vi "Set 1D Array Double Complex.vi"(5 "use temporary file? (F)":bool, 7 "column vector?":bool, 8 "error in":errorcluster, 9 "value":cdb[](array[numeric]), 10 "variable name":string, 11 "GOLPI ref. in":T1={"pipe handle"={"lv_proc.dll file path"=path "", "process instance handle"=[], "debug mode"=FALSE, "debug data"=[]}, "fast read timeout [ms]"=500, "fast read settle time [ms]"=10, "fast read to multiple [ms]"=1, "max elements per input line"=100, "slow read timeout [ms]"=5000, "stdin double format specifier"="%_16e", "max elements per stdout output column"=100, "console mode bitstream"=FALSE, "bitstream first read timeout [ms]"=1000, "bitstream read timeout [ms]"=50, "struct transfer possible"=FALSE, "matlab mode"=FALSE, "var pipe write timeout [ms]"=5000, "variable pipe mode"=FALSE, "variable pipe buffer size [Bytes]"=10000000, "variable pipe block size [Bytes]"=1000000} {"variable pipe block size [Bytes]" format="%.0p"; "variable pipe buffer size [Bytes]" format="%.0p"}) -> (0 "error out":errorcluster, 3 "GOLPI ref. out":T1={"pipe handle"={"lv_proc.dll file path"=path "", "process instance handle"=[], "debug mode"=FALSE, "debug data"=[]}, "fast read timeout [ms]"=500, "fast read settle time [ms]"=10, "fast read to multiple [ms]"=1, "max elements per input line"=100, "slow read timeout [ms]"=5000, "stdin double format specifier"="%_16e", "max elements per stdout output column"=100, "console mode bitstream"=FALSE, "bitstream first read timeout [ms]"=1000, "bitstream read timeout [ms]"=50, "struct transfer possible"=FALSE, "matlab mode"=FALSE, "var pipe write timeout [ms]"=5000, "variable pipe mode"=FALSE, "variable pipe buffer size [Bytes]"=10000000, "variable pipe block size [Bytes]"=1000000} {"variable pipe block size [Bytes]" format="%.0p"; "variable pipe buffer size [Bytes]" format="%.0p"})   [LabVIEW 2020, in "GOLPI library.lvlib"]
doc: "Part of polymorph Set Variable.vi"
uses:
  GOLPI library.lvlib
  Public/GOLPI reference Type Def.ctl
  LV Process source distribution/Pipe Handle.ctl
  LV Process source distribution/LV Process library.lvlib
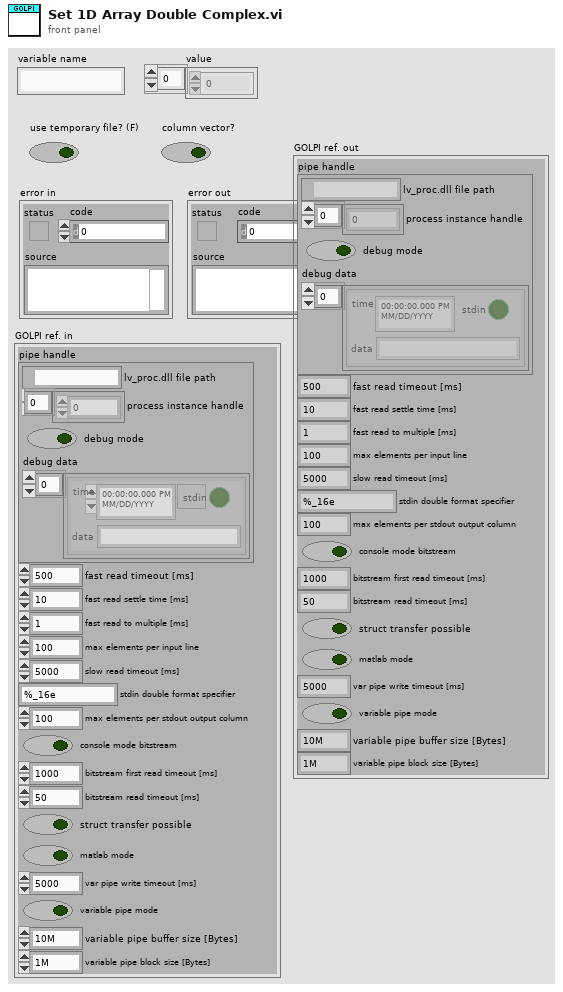
[diagram p1: front panel]
types:
  T1 = typedef "GOLPI library.lvlib/GOLPI reference Type Def.ctl" = cluster{"pipe handle":T2, "fast read timeout [ms]":u32, "fast read settle time [ms]":u32, "fast read to multiple [ms]":u32, "max elements per input line":u32, "slow read timeout [ms]":u32, "stdin double format specifier":string, "max elements per stdout output column":u32, "console mode bitstream":bool, "bitstream first read timeout [ms]":u32, "bitstream read timeout [ms]":u32, "struct transfer possible":bool, "matlab mode":bool, "var pipe write timeout [ms]":u32, "variable pipe mode":bool, "variable pipe buffer size [Bytes]":u32, "variable pipe block size [Bytes]":u32}
  T2 = typedef "LV Process library.lvlib/Pipe Handle.ctl" = cluster{"lv_proc.dll file path":path, "process instance handle":u32[], "debug mode":bool, "debug data":cluster{"time":timestamp, "stdin":bool, "data":string}[]}
  T3 = typedef "GOLPI library.lvlib/Transfer Mode.ctl" = enum16{"Matlab", "stdio", "temp file", "bitstream", "pipe"}
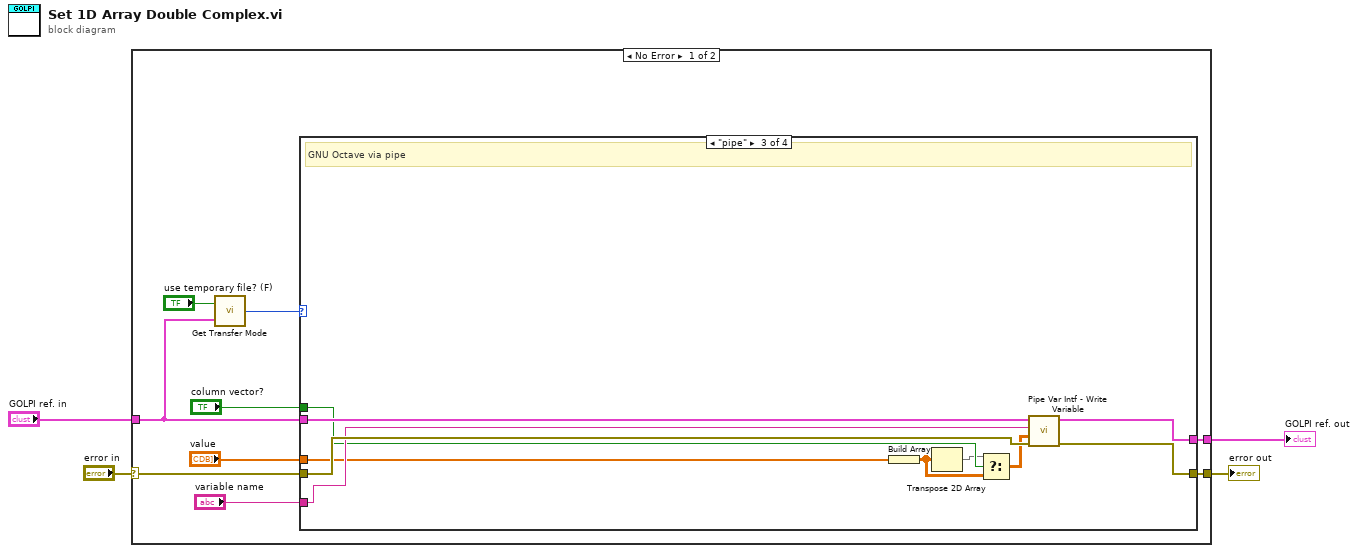
[diagram p0: block diagram]
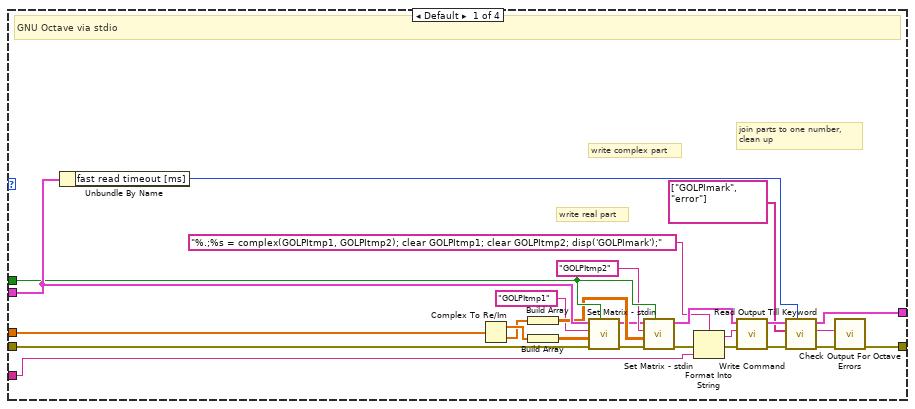
[diagram p2: hidden frame]
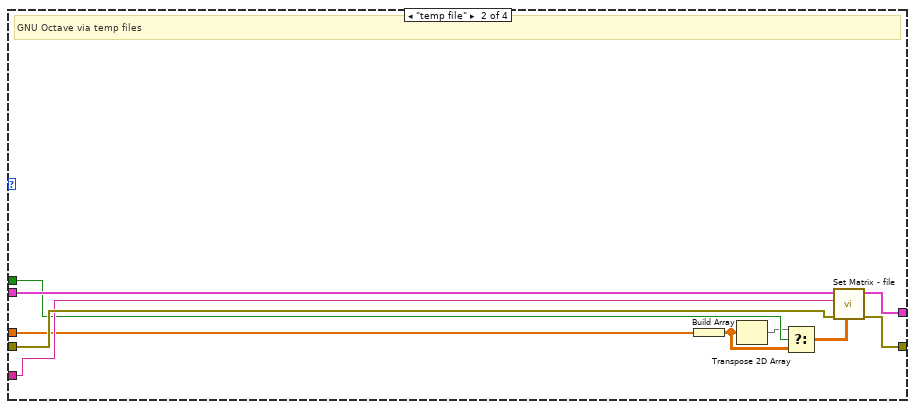
[diagram p3: hidden frame]
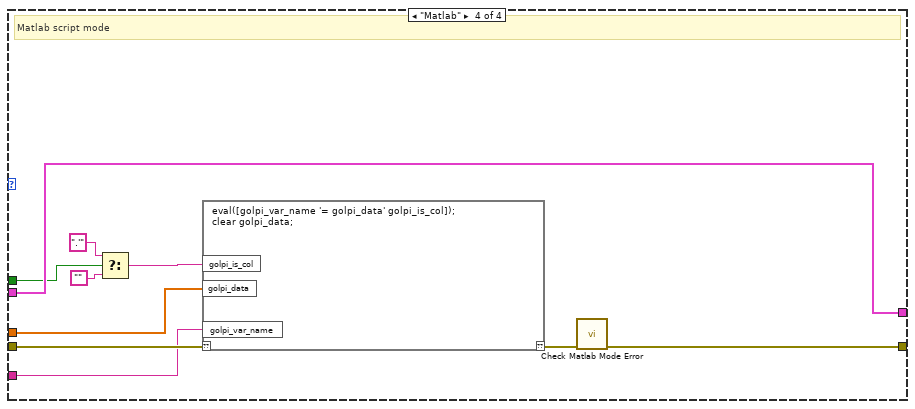
[diagram p4: hidden frame]
diagram:
  n1 = case shown="No Error" "error in" {
    selector: "error in" -> [w13 w71]
    tunnel: [w10 w71] -> w4
    tunnel: "GOLPI ref. in" -> [w7 w70]
    tunnel: [w11 w70] -> w1
    frame No Error {
      n2 = call "Get Transfer Mode.vi"("GOLPI ref."=w7, "use temporary file? (F)"="use temporary file? (F)") -> ("mode"=w5:T3)
      n3 = case shown="\"pipe\"" w5 {
        tunnel: w13 -> [w39 w49 w59 w69]
        tunnel: "variable name" -> [w38 w48 w58 w68]
        tunnel: [w37 w47 w57 w66] -> w11
        tunnel: [w36 w46 w56 w60] -> w10
        tunnel: w7 -> [w35 w45 w55 w66]
        tunnel: "column vector?" -> [w34 w44 w54 w63]
        tunnel: "value" -> [w33 w43 w53 w67]
        frame Default {
          # "join parts to one number,\nclean up"
          # "write complex part"
          # "write real part"
          # "GNU Octave via stdio"
          n4 = Unbundle By Name(w35) -> ("fast read timeout [ms]"=w15:u32)
          n5 = Complex To Re/Im(x + iy=w33) -> (x=w31:dbl[], y=w28:dbl[])
          n6 = Build Array(w28) -> (w29:dbl[][])
          n7 = Build Array(w31) -> (w32:dbl[][])
          n8 = call "Set Matrix - stdin.vi"("swap dimensions? (F)"=w34, "error in"=w39, "value"=w32, "variable name"="GOLPItmp1", "GOLPI ref. in"=w35) -> ("error out"=w27:errorcluster, "GOLPI ref. out"=w26:T1)  [unwired: 5 in]
          n9 = call "Set Matrix - stdin.vi"("swap dimensions? (F)"=w34, "error in"=w27, "value"=w29, "variable name"="GOLPItmp2", "GOLPI ref. in"=w26) -> ("error out"=w25:errorcluster, "GOLPI ref. out"=w24:T1)  [unwired: 5 in]
          n10 = Format Into String(format string="%.;%s = complex(GOLPItmp1, GOLPItmp2); clear GOLPItmp1; clear GOLPItmp2; disp('GOLPImark');" ("command"), error in=w25, w38) -> (resulting string=w22:string, error out=w23:errorcluster)  [unwired: 1 in]
          n11 = call "Write Command.vi"("error in"=w23, "command"=w22, "GOLPI ref. in"=w24) -> ("error out"=w20:errorcluster, "GOLPI ref. out"=w19:T1)  [unwired: 7 in]
          n12 = call "Read Output Till Keyword.vi"("timeout [ms]"=w15, "error in"=w20, "keywords"=string[] ["GOLPImark", "error"], "GOLPI ref. in"=w19) -> ("error out"=w17:errorcluster, "read buffer"=w16:string, "GOLPI ref. out"=w37:T1)  [unwired: 4 in, 1 out]
          n13 = call "Check Output For Octave Errors.vi"("error in"=w17, "read buffer"=w16) -> ("error out"=w36:errorcluster)  [unwired: 9 in]
        }
        frame "temp file" {
          # "GNU Octave via temp files"
          n14 = Build Array(w43) -> (w41:cdb[][])
          n15 = Transpose 2D Array(2D array=w41) -> (transposed array=w40:cdb[][])
          n16 = Select(t=w40, s=w44, f=w41) -> (s? t:f=w42:cdb[][])
          n17 = call "Set Matrix - file.vi"("cmplx double array"=w42, "error in (no error)"=w49, "variable name"=w48, "GOLPI ref. in"=w45) -> ("error out"=w46:errorcluster, "GOLPI ref. out"=w47:T1)  [unwired: 6 in]
        }
        frame "pipe" {
          # "GNU Octave via pipe"
          n18 = Build Array(w53) -> (w51:cdb[][])
          n19 = Transpose 2D Array(2D array=w51) -> (transposed array=w50:cdb[][])
          n20 = Select(t=w50, s=w54, f=w51) -> (s? t:f=w52:cdb[][])
          n21 = call "Pipe Var Intf - Write Variable.vi"("error in (no error)"=w59, "data in"=w52, "variable name"=w58, "GOLPI ref. in"=w55) -> ("error out"=w56:errorcluster, "GOLPI ref. out"=w57:T1)  [unwired: 6 in]
        }
        frame "Matlab" {
          # "Matlab script mode"
          n22 = Select(t=".'", s=w63, f="") -> (s? t:f=w62:string)
          n23 = script code="eval([golpi_var_name '= golpi_data' golpi_is_col]);\nclear golpi_data;"("??"=w69, "golpi_var_name"=w68, "golpi_data"=w67, "golpi_is_col"=w62) -> ("??"=w61:errorcluster)
          n24 = call "Check Matlab Mode Error.vi"("error in"=w61) -> ("error out"=w60:errorcluster)  [unwired: 10 in]
        }
      }
    }
    frame Error {
    }
  }
  "error out" <- w4
  "GOLPI ref. out" <- w1
